vi "08-cfp-pwm-timer.vi"() -> ()   [LabVIEW 2012]
uses:
  <vilib>/FieldPoint/Polymorphic Read.llb/FP Read (Float Array -IO).vi
  <vilib>/FieldPoint/Polymorphic Write.llb/FP Write (Float Array -IO).vi
panel:
  in  "?":enum32{"Главная", "Диагностика"}(tab)
  out "Обратный отсчет\nвремени, с":u8(slide) scale=0.0..25.0
  out "Номер отсчета":dbl
  out "Граница времени, с":dbl(knob)
  out "Поток\nвоздуха":dbl(knob) scale=0.0..100.0
  out "t, °C":dbl(slide) scale=25.0..50.0
  in  "Поток\nвоздуха, %":dbl(slide)=40.816326530612244 scale=0.0..100.0
  out "Задана t, °C":dbl(knob) scale=25.0..50.0
  in  "?":bool
  in  "FieldPoint IO Point (Output)":refnum<k21>="ivan\\NI-cFP2220-0165C974\\cFP-PWM-520 @3\\Channel 1"
  out "Write Error":errorcluster
  out "Read Error":errorcluster
  in  "FieldPoint IO Point":refnum<k21>="ivan\\NI-cFP2220-0165C974\\cFP-TC-120 @2\\Channel 1"
  # "Термостат:\nтемпературный режим"
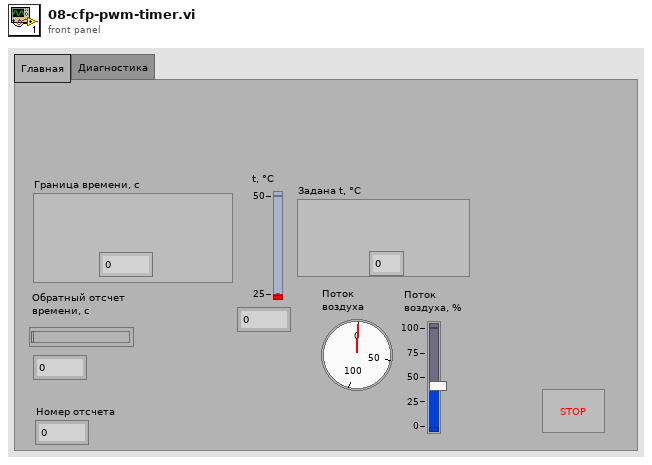
[diagram p1: front panel]
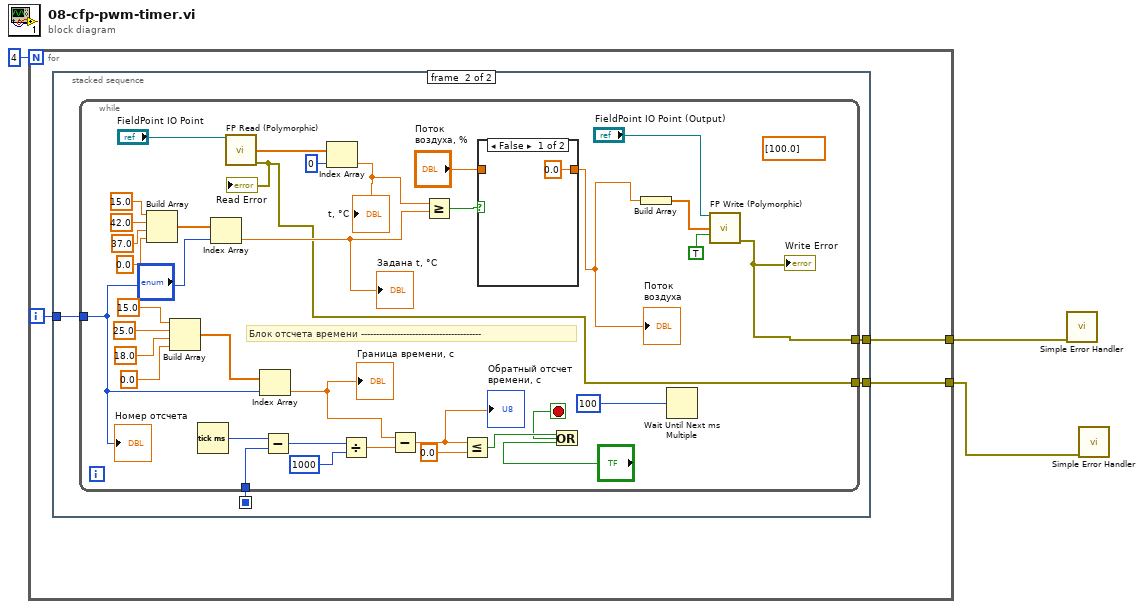
[diagram p0: block diagram]
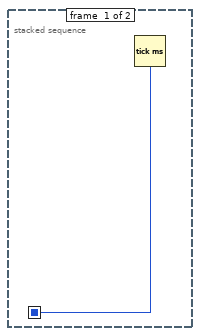
[diagram p2: hidden frame]
diagram:
  n1 = for {
    N: 4 -> [_]
    tunnel: [w5] -> w2
    tunnel: [w4] -> w1
    i -> [w6]
    n2 = stacked-sequence {
      seq-local: [w7 _] -> [_ w11]
      tunnel: w6 -> [_ w10]
      tunnel: [_ w9] -> w5
      tunnel: [_ w8] -> w4
      frame #0 {
        n3 = Tick Count (ms)() -> (millisecond timer value=w7:u32)
      }
      frame #1 {
        n4 = while {
          tunnel: w11 -> [w37]
          tunnel: w10 -> [w28]
          tunnel: [w15] -> w9
          tunnel: [w14] -> w8
          stop <- w17 stop-if-true
          (unwired) dbl[] [100.0] ("values")
          # "Блок отсчета времени ----------------------------------------"
          n5 = Build Array "Build Array"(15.0 ("element"), 42.0 ("element"), 37.0 ("element"), 0.0 ("element")) -> (w31:dbl[])
          n6 = Build Array "Build Array"(15.0 ("element"), 25.0 ("element"), 18.0 ("element"), 0.0 ("element")) -> (w39:dbl[])
          n7 = Tick Count (ms)() -> (millisecond timer value=w44:u32)
          n8 = Index Array "Index Array"(array=w31, index=w28) -> (element=w20:dbl)
          "Задана t, °C" <- w20
          n9 = call-poly <vilib>:"FP Read (Polymorphic).vi"("FieldPoint IO Point In"="FieldPoint IO Point") -> ("values"=w25:dbl[], "error out"=w14:errorcluster)  [unwired: 11 in, 2 out]
          "Read Error" <- w14
          n10 = Index Array "Index Array"(array=w39, index=w28) -> (element=w38:dbl)
          "Граница времени, с" <- w38
          n11 = Subtract(x=w44, y=w37) -> (x-y=w45:u32)
          n12 = Index Array(array=w25, index=0) -> (element=w21:dbl)
          "t, °C" <- w21
          n13 = Divide(x=w45, y=u32 1000) -> (x/y=w47:dbl)
          n14 = Subtract(x=w38, y=w47) -> (x-y=w27:dbl)
          "Обратный отсчет\nвремени, с" <- w27
          n15 = Greater Or Equal?(x=w21, y=w20) -> (x >= y?=w19:bool)
          n16 = Less Or Equal?(x=w27, y=0.0) -> (x <= y?=w18:bool)
          n17 = case shown="False" w19 {
            tunnel: "Поток\nвоздуха, %" -> [_ w49]
            tunnel: [0.0 w49] -> w12
            frame False {
            }
            frame True {
            }
          }
          "Поток\nвоздуха" <- w12
          n18 = Or(x=w18, y="?") -> (x .or. y?=w17:bool)
          n19 = Build Array "Build Array"(w12) -> (w13:dbl[])
          n20 = Wait Until Next ms Multiple(millisecond multiple=u32 100) -> ()  [unwired: 1 out]
          n21 = call-poly <vilib>:"FP Write (Polymorphic).vi"("FieldPoint IO Point In"="FieldPoint IO Point (Output)", "values"=w13, "on change (false)"=TRUE) -> ("error out"=w15:errorcluster)  [unwired: 10 in, 2 out]
          "Write Error" <- w15
          "Номер отсчета" <- w28
        }
      }
    }
  }
  n22 = call <vilib>:"Simple Error Handler.vi"("error in (no error)"=w2) -> ()  [unwired: 4 in, 5 out]
  n23 = call <vilib>:"Simple Error Handler.vi"("error in (no error)"=w1) -> ()  [unwired: 4 in, 5 out]
